vi "配置控件.vi"(4 "原备注":string, 5 "交互信息":string, 6 "关键字":string, 7 "原值":string) -> (0 "新备注":string, 1 "新值":string)   [LabVIEW 2020]
panel:
  in  "备注":string
  in  "确定":bool
  in  "取消":bool
  in  "选项卡":T1(tab)
  in  "列表":string
  in  "元素":string
  in  "变量/常量":string
  in  "提示":u16(ring) items=["端口"]
  in  "备选信息":string(combo)
  in  "out":string
  in  "比较符号":string(combo)
  in  "逻辑运算":string(combo)
  in  "数学运算":string(combo)
  # "："
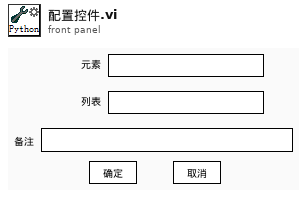
[diagram p1: front panel]
types:
  T1 = enum32{"for", "in", "out", "compare", "logic", "math"}
  T2 = typedef "LVComboBoxStrsAndValuesArrayTypeDef.ctl" = cluster{"String":string, "Value":string}[]
  T3 = typedef "eventvkey.ctl" = enum16{"ASCII", "Enter", "Return", "Shift", "Ctrl", "Alt", "Cmd", "Opt", "Caps", "NumLock", "Clear", "Break", "Up", "Down", "Left", "Right", "Insert", "Delete", "Home", "End", "PageUp", "PageDown", "Escape", "Help", "Pause", "ScrollLock", "F1", "F2", "F3", "F4", "F5", "F6", "F7", "F8", "F9", "F10", "F11", "F12", "F13", "F14", "F15", "F16", "F17", "F18", "F19", "F20", "F21", "F22", "F23", "F24", "Play", "VolumeUp", "VolumeDown", "Mute", "Two Byte Char"}
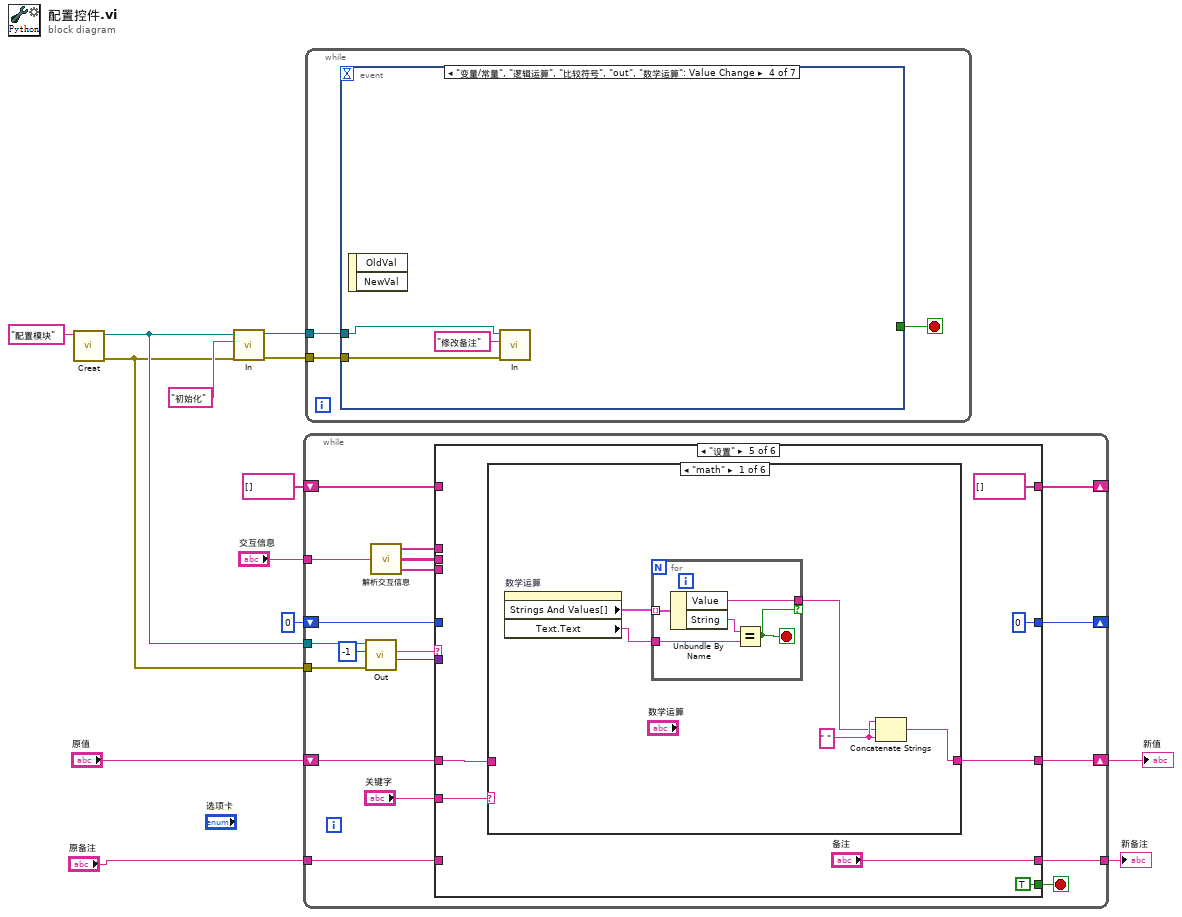
[diagram p0: block diagram]
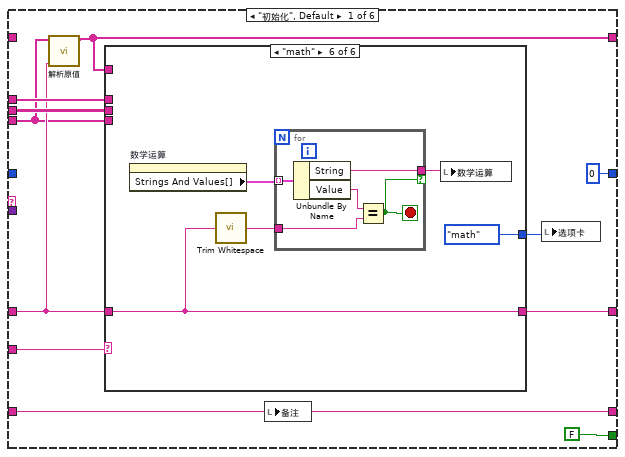
[diagram p2: hidden frame]
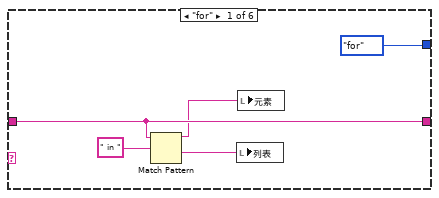
[diagram p3: hidden frame]
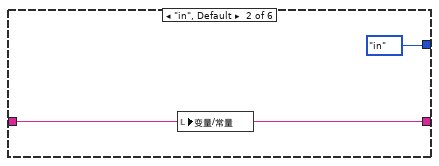
[diagram p4: hidden frame]
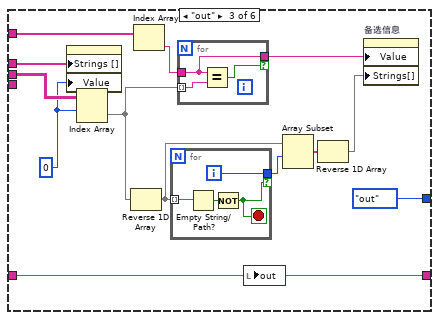
[diagram p5: hidden frame]
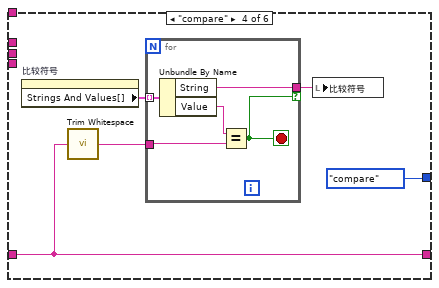
[diagram p6: hidden frame]
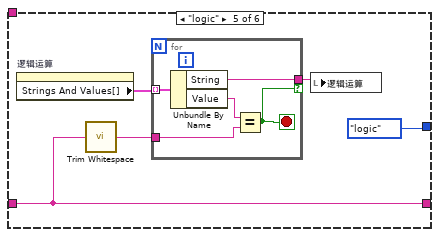
[diagram p7: hidden frame]
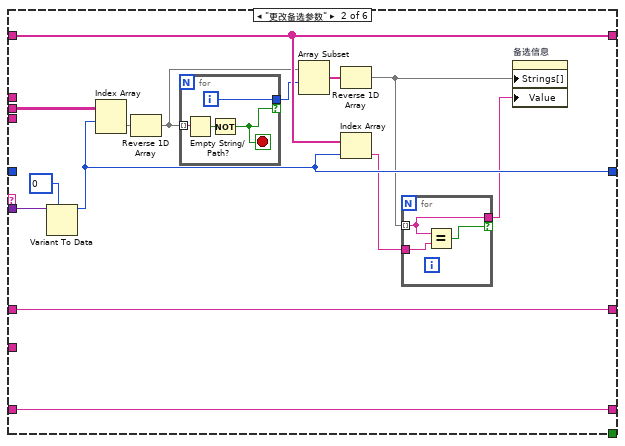
[diagram p8: hidden frame]
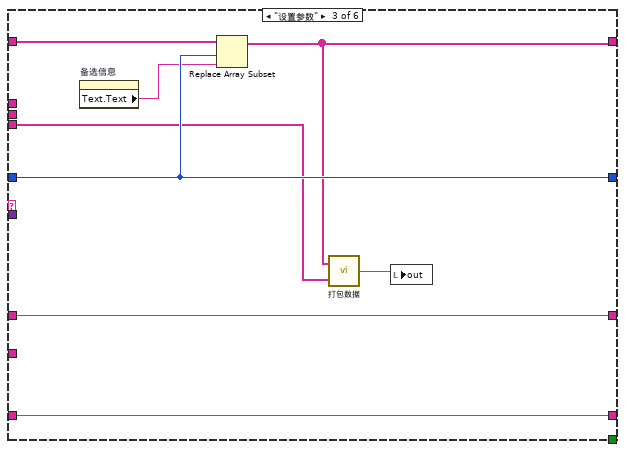
[diagram p9: hidden frame]
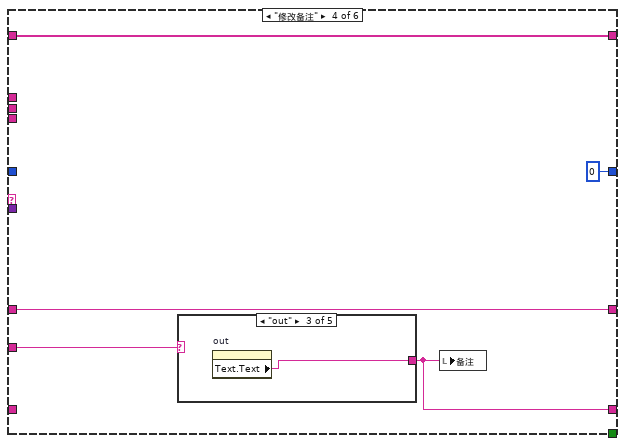
[diagram p10: hidden frame]
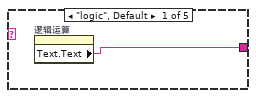
[diagram p11: hidden frame]
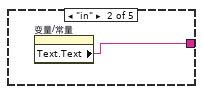
[diagram p12: hidden frame]
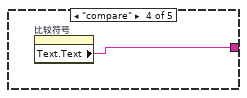
[diagram p13: hidden frame]
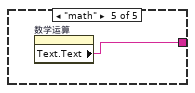
[diagram p14: hidden frame]
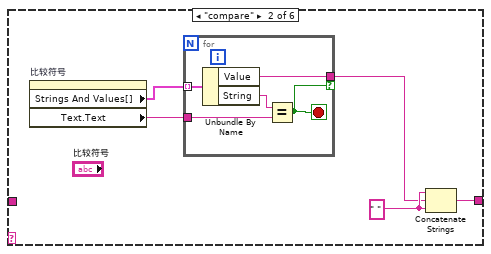
[diagram p15: hidden frame]
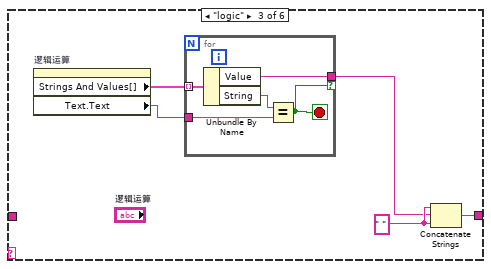
[diagram p16: hidden frame]
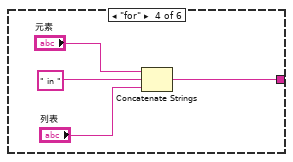
[diagram p17: hidden frame]
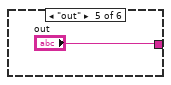
[diagram p18: hidden frame]
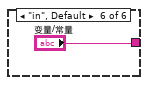
[diagram p19: hidden frame]
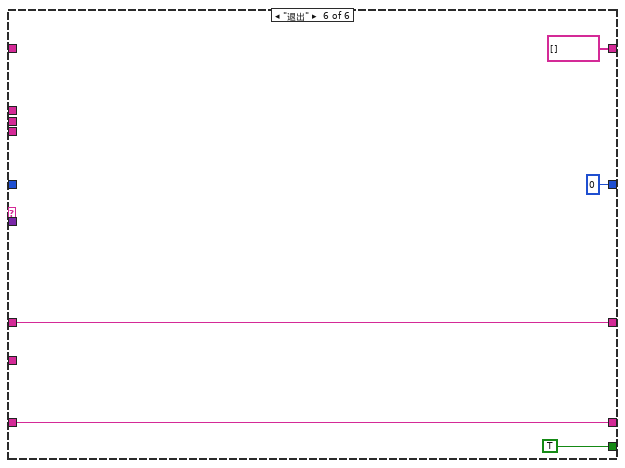
[diagram p20: hidden frame]
diagram:
  n1 = call "Creat.vi"("名称"="配置模块") -> ("错误输出"=w6:errorcluster, "队列输出"=w7:refnum<queue>)  [unwired: 9 in]
  n2 = call "In.vi"("错误输入"=w6, "指令"="初始化", "队列"=w7) -> ("错误输出"=w9:errorcluster, "队列输出"=w8:refnum<queue>)  [unwired: 7 in]
  n3 = while {
    shift-right: [w31] -> w11
    shift-left: "原值" -> [w32]
    tunnel: w7 -> [w28]
    tunnel: w6 -> [w27]
    tunnel: "交互信息" -> [w23]
    shift-right: [w19] -> _
    shift-left: string[] [] ("提示") -> [w18]
    shift-right: [w17] -> _
    shift-left: u16 0 ("提示") -> [w16]
    tunnel: [w15] -> w1
    tunnel: "原备注" -> [w14]
    stop <- w30 stop-if-true
    n4 = call "Out.vi"("错误输入"=w27, "超时毫秒(-1)"=-1, "队列"=w28) -> ("数据"=w24:variant, "指令"=w26:string)  [unwired: 5 in, 2 out]
    n5 = call "解析交互信息.vi"("交互信息"=w23) -> ("提示"=w22:string[], "备选信息"=w21:string[][], "补充信息"=w20:string[])  [unwired: 4 in]
    n6 = case shown="\"设置\"" w26 {
      tunnel: w32 -> [w37 w112 w123 w132 w143 w184]
      tunnel: "关键字" -> [w43 _ _ w130 w146 _]
      tunnel: [w42 w112 w123 w132 w145 w184] -> w31
      tunnel: [FALSE _ _ _ TRUE TRUE] -> w30
      tunnel: w24 -> [_ w114 _ _ _ _]
      tunnel: w22 -> [w39 _ _ _ _ _]
      tunnel: w21 -> [w40 w113 _ _ _ _]
      tunnel: w20 -> [w36 _ w126 _ _ _]
      tunnel: [w35 w110 w127 w133 string[] [] ("提示") string[] [] ("提示")] -> w19
      tunnel: w18 -> [_ w110 w129 w133 _ _]
      tunnel: [u16 0 ("提示") w109 w128 u16 0 ("提示") u16 0 ("提示") u16 0 ("提示")] -> w17
      tunnel: w16 -> [_ _ w128 _ _ _]
      tunnel: [w34 w106 w124 w131 "备注" w183] -> w15
      tunnel: w14 -> [w34 w106 w124 _ _ w183]
      frame "初始化", Default {
        n7 = call "解析原值.vi"("原值"=w37, "补充信息"=w36) -> ("参数"=w35:string[])  [unwired: 9 in]
        n8 = case shown="\"math\"" w43 {
          tunnel: w37 -> [w48 w50 w62 w74 w85 w93]
          tunnel: [w48 w50 w62 w74 w85 w93] -> w42
          tunnel: w39 -> [_ _ w63 _ _ _]
          tunnel: w40 -> [_ _ w61 _ _ _]
          tunnel: w36 -> [_ _ _ _ _ _]
          tunnel: w35 -> [_ _ w58 _ _ _]
          tunnel: [T1."for" ("选项卡") T1."in" ("选项卡") T1."out" ("选项卡") T1."compare" ("选项卡") T1."logic" ("选项卡") T1."math" ("选项卡")] -> w33
          frame "for" {
            n9 = Match Pattern(string=w48, regular expression=" in " ("字符串")) -> (before substring=w47:string, after substring=w46:string)  [unwired: 1 in, 2 out]
            n10 = local write "列表"(w46) -> ()
            n11 = local write "元素"(w47) -> ()
          }
          frame "in", Default {
            n12 = local write "变量/常量"(w50) -> ()
          }
          frame "out" {
            w60 = u16 0
            n13 = property on="提示" class="Ring (strict)"("Strings []"=w63, "Value"=w60) -> ()  [unwired: 2 in, 2 out]
            n14 = Index Array(array=w61, index (row)=w60) -> (element=w53:string[])  [unwired: 1 in]
            n15 = Reverse 1D Array(array=w53) -> (reversed array=w56:string[])
            n16 = Index Array(array=w58) -> (element=w57:string)  [unwired: 1 in]
            n17 = for {
              tunnel: w56 -> [w67] mode=indexing
              tunnel: [w66] -> w55 if=w64
              i -> [w66]
              stop <- w64 stop-if-true
              n18 = Empty String/Path?(string/path=w67) -> (empty?=w65:bool)
              n19 = Not(x=w65) -> (.not. x?=w64:bool)
            }
            n20 = for {
              tunnel: w57 -> [w68]
              tunnel: w53 -> [w70] mode=indexing
              tunnel: [w68] -> w59 if=w69
              n21 = Equal?(x=w68, y=w70) -> (x = y?=w69:bool)
            }
            n22 = local write "out"(w62) -> ()
            n23 = Array Subset(array=w56, index=w55) -> (w54:string[])  [unwired: 1 in]
            n24 = Reverse 1D Array(array=w54) -> (reversed array=w52:string[])
            n25 = property on="备选信息" class="CmbBox"("Value"=w59, "Strings[]"=w52) -> ()  [unwired: 2 in, 2 out]
          }
          frame "compare" {
            n26 = property on="比较符号" class="CmbBox"() -> ("Strings And Values[]"=w75:T2)  [unwired: 2 in, 2 out]
            n27 = call <vilib>:"Trim Whitespace.vi"("string"=w74) -> ("trimmed string"=w73:string)  [unwired: 1 in]
            n28 = for {
              tunnel: w73 -> [w80]
              tunnel: w75 -> [w79] mode=indexing
              tunnel: [w77] -> w72 if=w76
              stop <- w76 stop-if-true
              n29 = Unbundle By Name(w79) -> ("String"=w77:string, "Value"=w78:string)
              n30 = Equal?(x=w78, y=w80) -> (x = y?=w76:bool)
            }
            n31 = local write "比较符号"(w72) -> ()
          }
          frame "logic" {
            n32 = property on="逻辑运算" class="CmbBox"() -> ("Strings And Values[]"=w84:T2)  [unwired: 2 in, 2 out]
            n33 = call <vilib>:"Trim Whitespace.vi"("string"=w85) -> ("trimmed string"=w83:string)  [unwired: 1 in]
            n34 = for {
              tunnel: w83 -> [w90]
              tunnel: w84 -> [w89] mode=indexing
              tunnel: [w87] -> w82 if=w86
              stop <- w86 stop-if-true
              n35 = Unbundle By Name(w89) -> ("String"=w87:string, "Value"=w88:string)
              n36 = Equal?(x=w88, y=w90) -> (x = y?=w86:bool)
            }
            n37 = local write "逻辑运算"(w82) -> ()
          }
          frame "math" {
            n38 = property on="数学运算" class="CmbBox"() -> ("Strings And Values[]"=w94:T2)  [unwired: 2 in, 2 out]
            n39 = call <vilib>:"Trim Whitespace.vi"("string"=w93) -> ("trimmed string"=w92:string)  [unwired: 1 in]
            n40 = for {
              tunnel: w92 -> [w100]
              tunnel: w94 -> [w99] mode=indexing
              tunnel: [w97] -> w91 if=w96
              stop <- w96 stop-if-true
              n41 = Unbundle By Name(w99) -> ("String"=w97:string, "Value"=w98:string)
              n42 = Equal?(x=w98, y=w100) -> (x = y?=w96:bool)
            }
            n43 = local write "数学运算"(w91) -> ()
          }
        }
        n44 = local write "备注"(w34) -> ()
        n45 = local write "选项卡"(w33) -> ()
      }
      frame "更改备选参数" {
        w111 = u16 0 items=[""] ("提示")
        n46 = Variant To Data(type=w111, Variant=w114) -> (data=w109:u16)  [unwired: 1 in, 1 out]
        n47 = Index Array(array=w113, index (row)=w109) -> (element=w105:string[])  [unwired: 1 in]
        n48 = Reverse 1D Array(array=w105) -> (reversed array=w104:string[])
        n49 = for {
          tunnel: w104 -> [w118] mode=indexing
          tunnel: [w117] -> w103 if=w115
          i -> [w117]
          stop <- w115 stop-if-true
          n50 = Empty String/Path?(string/path=w118) -> (empty?=w116:bool)
          n51 = Not(x=w116) -> (.not. x?=w115:bool)
        }
        n52 = Array Subset(array=w104, index=w103) -> (w102:string[])  [unwired: 1 in]
        n53 = Reverse 1D Array(array=w102) -> (reversed array=w101:string[])
        n54 = Index Array(array=w110, index=w109) -> (element=w108:string)
        n55 = for {
          tunnel: w108 -> [w121]
          tunnel: w101 -> [w119] mode=indexing
          tunnel: [w119] -> w107 if=w120
          n56 = Equal?(x=w119, y=w121) -> (x = y?=w120:bool)
        }
        n57 = property on="备选信息" class="CmbBox"("Strings[]"=w101, "Value"=w107) -> ()  [unwired: 2 in, 2 out]
      }
      frame "设置参数" {
        n58 = property on="备选信息" class="CmbBox"() -> ("Text.Text"=w125:string)  [unwired: 2 in, 2 out]
        n59 = Replace Array Subset(array=w129, new element=w125, index=w128) -> (w127:string[])
        n60 = call "打包数据.vi"("补充信息"=w126, "备选信息"=w127) -> ("语句"=w122:string)
        n61 = local write "out"(w122) -> ()
      }
      frame "修改备注" {
        n62 = case shown="\"out\"" w130 {
          tunnel: [w135 w136 w137 w138 w139] -> w131
          frame "logic", Default {
            n63 = property on="逻辑运算" class="CmbBox"() -> ("Text.Text"=w135:string)  [unwired: 2 in, 2 out]
          }
          frame "in" {
            n64 = property on="变量/常量" class="Str"() -> ("Text.Text"=w136:string)  [unwired: 2 in, 2 out]
          }
          frame "out" {
            n65 = property on="out" class="Str"() -> ("Text.Text"=w137:string)  [unwired: 2 in, 2 out]
          }
          frame "compare" {
            n66 = property on="比较符号" class="CmbBox"() -> ("Text.Text"=w138:string)  [unwired: 2 in, 2 out]
          }
          frame "math" {
            n67 = property on="数学运算" class="CmbBox"() -> ("Text.Text"=w139:string)  [unwired: 2 in, 2 out]
          }
        }
        n68 = local write "备注"(w131) -> ()
      }
      frame "设置" {
        n69 = case shown="\"math\"" w146 {
          tunnel: [w151 w161 w171 w177 "out" "变量/常量"] -> w145
          tunnel: w143 -> [_ _ _ _ _ _]
          frame "math" {
            w150 = " " ("字符串")
            n70 = property on="数学运算" class="CmbBox"() -> ("Strings And Values[]"=w149:T2, "Text.Text"=w148:string)  [unwired: 2 in, 2 out]
            n71 = for {
              tunnel: w148 -> [w156]
              tunnel: w149 -> [w155] mode=indexing
              tunnel: [w153] -> w147 if=w152
              stop <- w152 stop-if-true
              n72 = Unbundle By Name(w155) -> ("Value"=w153:string, "String"=w154:string)
              n73 = Equal?(x=w154, y=w156) -> (x = y?=w152:bool)
            }
            n74 = Concatenate Strings(w150, w147, w150) -> (w151:string)
          }
          frame "compare" {
            w160 = " " ("字符串")
            n75 = property on="比较符号" class="CmbBox"() -> ("Strings And Values[]"=w159:T2, "Text.Text"=w158:string)  [unwired: 2 in, 2 out]
            n76 = for {
              tunnel: w158 -> [w166]
              tunnel: w159 -> [w165] mode=indexing
              tunnel: [w163] -> w157 if=w162
              stop <- w162 stop-if-true
              n77 = Unbundle By Name(w165) -> ("Value"=w163:string, "String"=w164:string)
              n78 = Equal?(x=w164, y=w166) -> (x = y?=w162:bool)
            }
            n79 = Concatenate Strings(w160, w157, w160) -> (w161:string)
          }
          frame "logic" {
            w170 = " " ("字符串")
            n80 = property on="逻辑运算" class="CmbBox"() -> ("Strings And Values[]"=w168:T2, "Text.Text"=w167:string)  [unwired: 2 in, 2 out]
            n81 = for {
              tunnel: w167 -> [w176]
              tunnel: w168 -> [w175] mode=indexing
              tunnel: [w173] -> w169 if=w172
              stop <- w172 stop-if-true
              n82 = Unbundle By Name(w175) -> ("Value"=w173:string, "String"=w174:string)
              n83 = Equal?(x=w174, y=w176) -> (x = y?=w172:bool)
            }
            n84 = Concatenate Strings(w170, w169, w170) -> (w171:string)
          }
          frame "for" {
            n85 = Concatenate Strings("元素", " in " ("字符串"), "列表") -> (w177:string)
          }
          frame "out" {
          }
          frame "in", Default {
          }
        }
      }
      frame "退出" {
      }
    }
  }
  "新值" <- w11
  "新备注" <- w1
  n86 = while {
    tunnel: w8 -> [w189]
    tunnel: w9 -> [w188]
    stop <- w190 stop-if-true
    n87 = event shown="[3] \"变量/常量\", \"逻辑运算\", \"比较符号\", \"out\", \"数学运算\": Value Change" {
      selector: _ -> [_ _ _ _ _ _ _]
      dyn-events: _ -> [_ _ _ _ _ _ _]
      timeout: _ -> [_ _ _ _ _ _ _]
      tunnel: [w193 _ _ _ TRUE TRUE TRUE] -> w190
      tunnel: w189 -> [w192 w202 w206 w208 w211 w216 w219]
      tunnel: w188 -> [w191 w201 w205 w207 w210 w214 w218]
      event Key Down {
        n88 = event-data() -> ("VKey"=w194:T3)  [unwired: 1 in]
        n89 = case shown="\"Shift\", Default" w194 {
          tunnel: [_ TRUE] -> w193
          tunnel: w192 -> [_ w197]
          tunnel: w191 -> [_ w196]
          frame "Shift", Default {
          }
          frame "Return" {
            n90 = call "In.vi"("错误输入"=w196, "指令"="设置", "队列"=w197) -> ()  [unwired: 7 in, 2 out]
          }
        }
      }
      event "提示": Value Change {
        n91 = event-data() -> ("NewVal"=w199:u16)  [unwired: 1 in]
        n92 = To Variant(anything=w199) -> (Variant=w200:variant)
        n93 = call "In.vi"("错误输入"=w201, "数据"=w200, "指令"="更改备选参数", "队列"=w202) -> ()  [unwired: 6 in, 2 out]
      }
      event "备选信息": Value Change; "备选信息": Mouse Down; "备选信息": Mouse Up {
        n94 = event-data() -> ()  [unwired: 1 in, 1 out]
        n95 = call "In.vi"("错误输入"=w205, "指令"="设置参数", "队列"=w206) -> ()  [unwired: 7 in, 2 out]
      }
      event "变量/常量", "逻辑运算", "比较符号", "out", "数学运算": Value Change {
        n96 = event-data() -> ()  [unwired: 1 in, 2 out]
        n97 = call "In.vi"("错误输入"=w207, "指令"="修改备注", "队列"=w208) -> ()  [unwired: 7 in, 2 out]
      }
      event "确定": Mouse Down {
        n98 = event-data() -> ()  [unwired: 1 in, 1 out]
        n99 = call "In.vi"("错误输入"=w210, "指令"="设置", "队列"=w211) -> ()  [unwired: 7 in, 2 out]
      }
      event Panel Close {
        n100 = event-data() -> ()  [unwired: 1 in, 1 out]
        n101 = call "In.vi"("错误输入"=w214, "指令"="退出", "队列"=w216) -> ()  [unwired: 7 in, 2 out]
      }
      event "取消": Mouse Down {
        n102 = event-data() -> ()  [unwired: 1 in, 1 out]
        n103 = call "In.vi"("错误输入"=w218, "指令"="退出", "队列"=w219) -> ()  [unwired: 7 in, 2 out]
      }
    }
  }
